vi "Test Levels.vi"() -> ()   [LabVIEW 2020]
uses:
  VoiceMeeterRemote/Voicemeeter Type.ctl
  VoiceMeeterRemote/VoiceMeeterRemote/VoiceMeeterRemote.lvclass
  VoiceMeeterRemote/VoiceMeeterRemote.lvlib
panel:
  out "Type":T1
  out "A2 Right":sgl(slide) scale=0.0..1.0
  out "A2 Left":sgl(slide) scale=0.0..1.0
  out "Chart":sgl(graph)
  in  "stop":bool
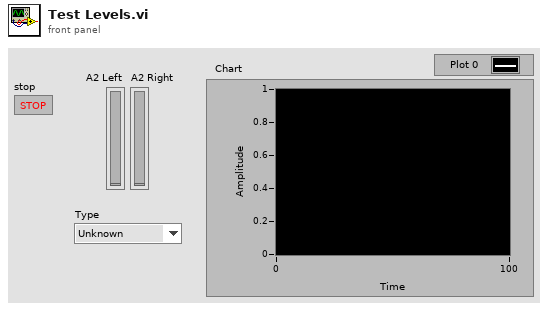
[diagram p1: front panel]
types:
  T1 = typedef "VoiceMeeterRemote.lvlib/Voicemeeter Type.ctl" = enum16{"Unknown", "Voicemeeter", "Banana", "Potato", "Potato x64"}
  T2 = typedef "VoiceMeeterRemote.lvlib/Levels.ctl" = cluster{"Input Pre Fader":T3[], "Input Post Fader":T3[], "Input Post Mute":T3[], "Output":T3[]}
  T3 = typedef "VoiceMeeterRemote.lvlib/Device Channels.ctl" = cluster{"Values":sgl[]}
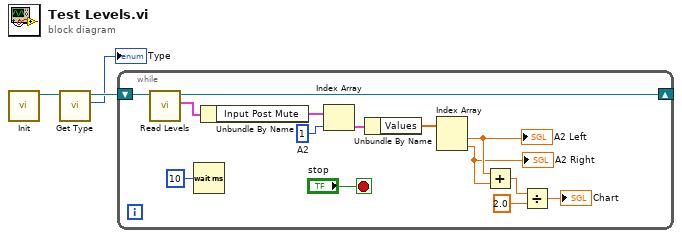
[diagram p0: block diagram]
diagram:
  n1 = call "Init.vi"() -> ("VoiceMeeterRemote out"=w3:refnum<class "VoiceMeeterRemote.lvclass">)  [unwired: 9 in, 2 out]
  n2 = call "Get Type.vi"("VoiceMeeterRemote in"=w3) -> ("Type"=→"Type":T1, "VoiceMeeterRemote out"=w2:refnum<class "VoiceMeeterRemote.lvclass">)  [unwired: 8 in, 1 out]
  n3 = while {
    shift-right: [w15] -> _
    shift-left: w2 -> [w17]
    stop <- "stop" stop-if-true
    w11 = 1  # A2
    n4 = call "Read Levels.vi"("VoiceMeeterRemote in"=w17) -> ("Levels"=w13:T2, "VoiceMeeterRemote out"=w15:refnum<class "VoiceMeeterRemote.lvclass">)  [unwired: 8 in, 1 out]
    n5 = Wait (ms)(milliseconds to wait=u32 10) -> ()  [unwired: 1 out]
    n6 = Unbundle By Name(w13) -> ("Input Post Mute"=w12:T3[])
    n7 = Index Array(array=w12, index=w11) -> (element=w10:T3)
    n8 = Unbundle By Name(w10) -> ("Values"=w9:sgl[])
    n9 = Index Array(array=w9) -> (element #1=w8:sgl, element #2=w7:sgl)  [unwired: 2 in]
    "A2 Left" <- w8
    "A2 Right" <- w7
    n10 = Add(x=w8, y=w7) -> (x+y=w6:sgl)
    n11 = Divide(x=w6, y=sgl 2.0) -> (x/y=→"Chart":sgl)
  }
